vi "enableOut.vi"(8 "error in (no error)":errorcluster) -> (0 "error out":errorcluster, 3 "DS360 out":refnum<class "DS360.lvclass">)   [LabVIEW 2019, in "DS360.lvclass"]
uses:
  DS360.lvclass
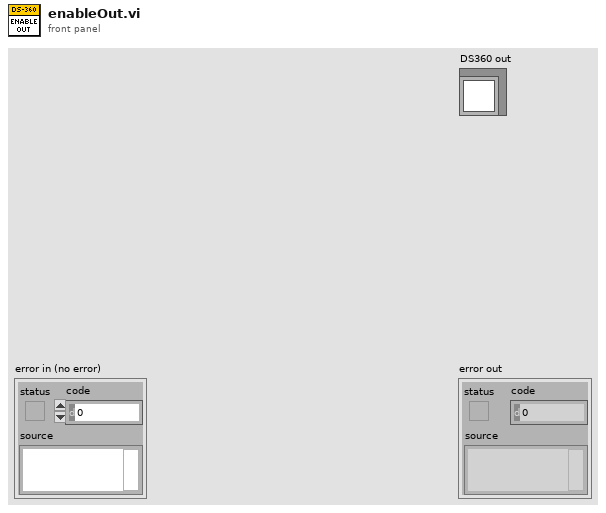
[diagram p1: front panel]
types:
  T1 = cluster{"error":bool, "code":i32, "source":string}
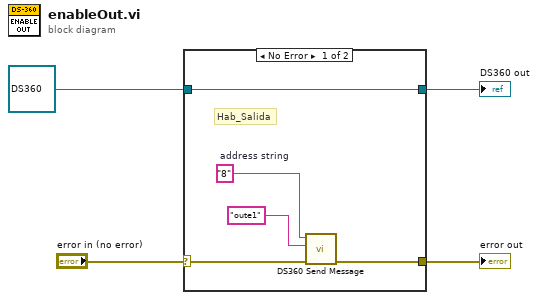
[diagram p0: block diagram]
diagram:
  n1 = case shown="No Error" "error in (no error)" {
    selector: "error in (no error)" -> [w6 w11]
    tunnel: [w5 w11] -> w3
    tunnel: [w9 w10] -> w1
    tunnel: refnum<class "DS360.lvclass"> refnum ("DS360 in") -> [w9 w10]
    frame No Error {
      w7 = "8"  # address string
      # "Hab_Salida"
      n2 = call <instrlib>:"DS360 Send Message.vi"("address string"=w7, "write buffer"="oute1", "error in"=w6) -> ("error out"=w5:T1)  [unwired: 3 in, 3 out]
    }
    frame Error {
    }
  }
  "error out" <- w3
  "DS360 out" <- w1
